vi "ADCP_read_symbol_file.vi"(8 "error in (no error)":errorcluster, 10 "Symbol File Path":path, 11 "ADCP in":refnum<class "ADCP.lvclass">) -> (0 "error out":errorcluster, 1 "Data Packets":T2(array[cluster]), 2 "Parameters":T3(array[cluster]), 3 "ADCP out":refnum<class "ADCP.lvclass">)   [LabVIEW 2017, in "ADCP.lvclass"]
uses:
  ADCP.lvclass
  ADCP_Data_Packet_Transmit_Mode.ctl
  ADCP.lvclass/ADCP.ctl
  <vilib>/Utility/file.llb/Read Delimited Spreadsheet (string).vi
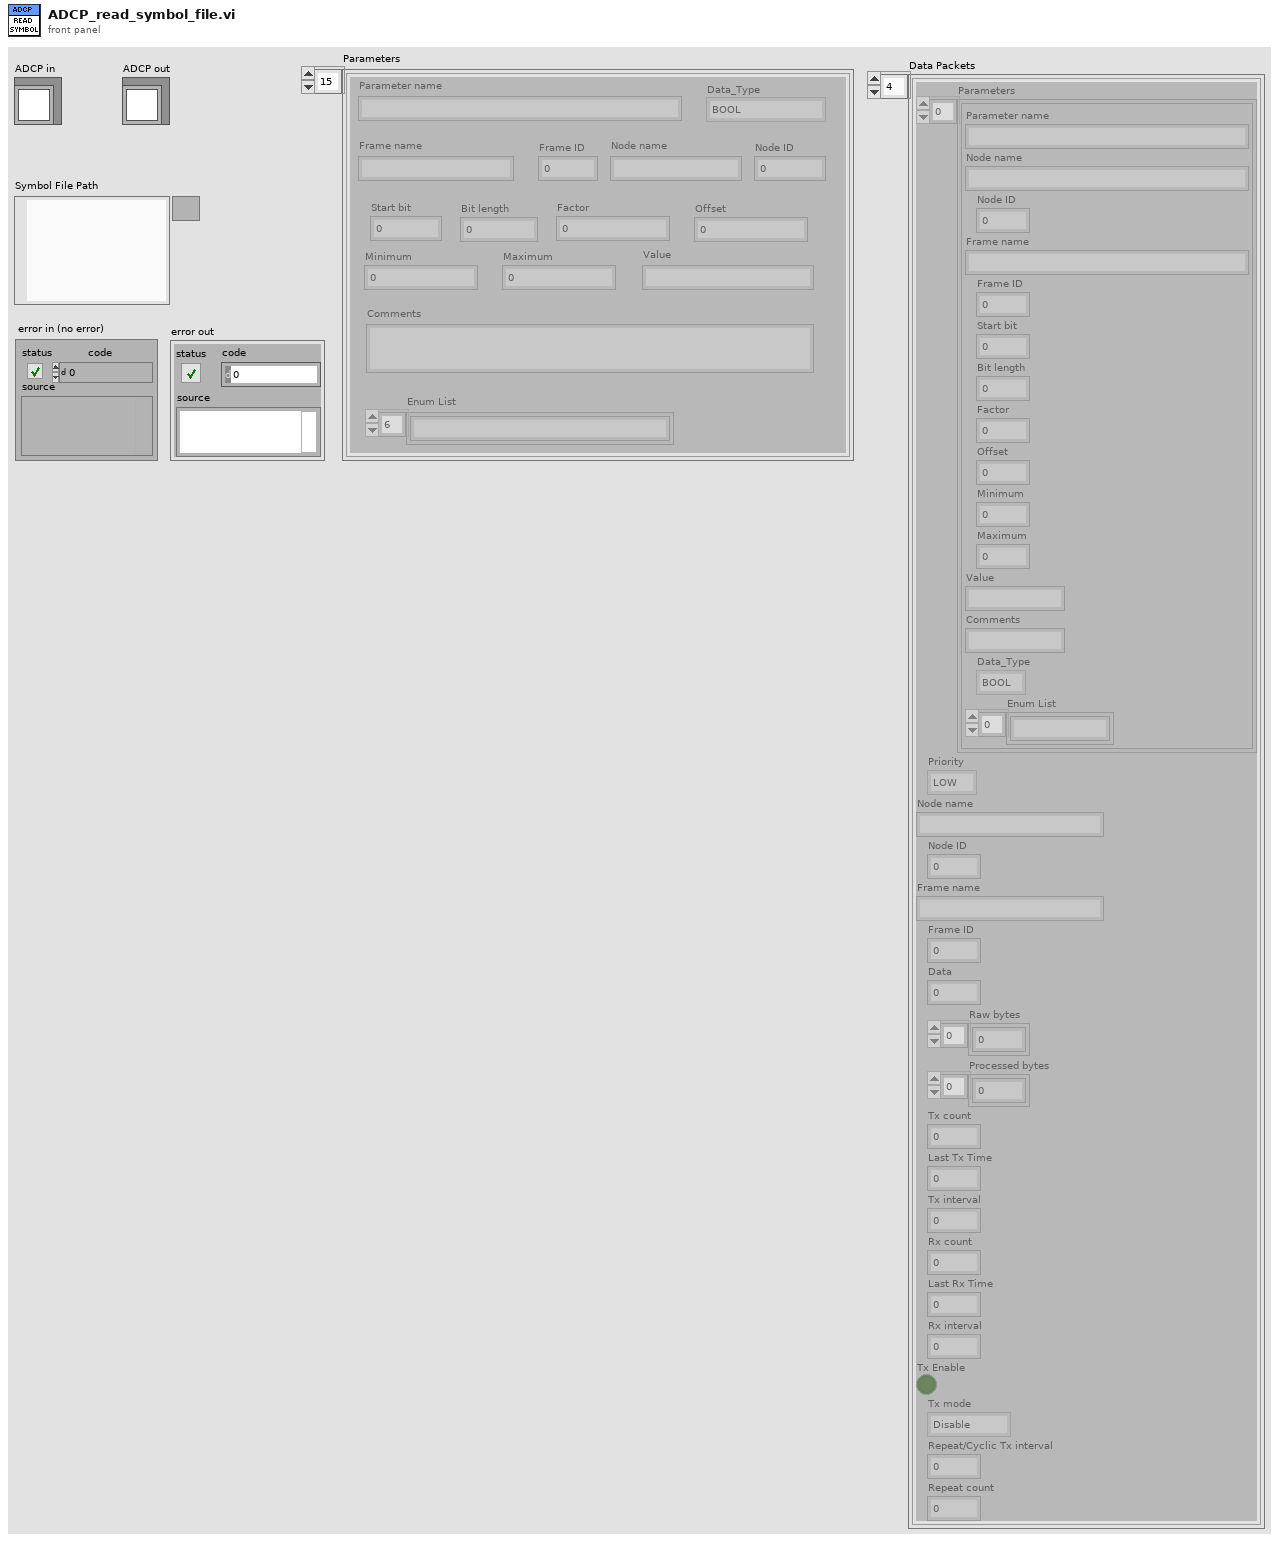
[diagram p1: front panel]
types:
  T1 = typedef "ADCP.lvclass/ADCP_Data_Packet_Transmit_Mode.ctl" = enum16{"Disable", "Single", "Cyclic", "Repeat"}
  T2 = cluster{"Parameters":cluster{"Parameter name":string, "Node name":string, "Node ID":u8, "Frame name":string, "Frame ID":u8, "Start bit":u32, "Bit length":u32, "Factor":dbl, "Offset":dbl, "Minimum":dbl, "Maximum":dbl, "Value":string, "Comments":string, "Data_Type":enum16{"BOOL", "UNSIGNED", "SIGNED", "FLOAT32", "ENUM"}, "Enum List":string[]}[], "Priority":enum16{"LOW", "HIGH"}, "Node name":string, "Node ID":u8, "Frame name":string, "Frame ID":u8, "Data":u32, "Raw bytes":u8[], "Processed bytes":u8[], "Tx count":i32, "Last Tx Time":u32, "Tx interval":u32, "Rx count":i32, "Last Rx Time":u32, "Rx interval":u32, "Tx Enable":bool, "Tx mode":T1, "Repeat/Cyclic Tx interval":u32, "Repeat count":u16}[]
  T3 = cluster{"Parameter name":string, "Node name":string, "Node ID":u8, "Frame name":string, "Frame ID":u8, "Start bit":u32, "Bit length":u32, "Factor":dbl, "Offset":dbl, "Minimum":dbl, "Maximum":dbl, "Value":string, "Comments":string, "Data_Type":enum16{"BOOL", "UNSIGNED", "SIGNED", "FLOAT32", "ENUM"}, "Enum List":string[]}[]
  T4 = cluster{"Parameter name":string, "Node name":string, "Node ID":u8, "Frame name":string, "Frame ID":u8, "Start bit":u32, "Bit length":u32, "Factor":dbl, "Offset":dbl, "Minimum":dbl, "Maximum":dbl, "Value":string, "Comments":string, "Data_Type":enum16{"BOOL", "UNSIGNED", "SIGNED", "FLOAT32", "ENUM"}, "Enum List":string[]}
  T5 = enum16{"BOOL", "UNSIGNED", "SIGNED", "FLOAT32", "ENUM"}
  T6 = cluster{"Parameters":cluster{"Parameter name":string, "Node name":string, "Node ID":u8, "Frame name":string, "Frame ID":u8, "Start bit":u32, "Bit length":u32, "Factor":dbl, "Offset":dbl, "Minimum":dbl, "Maximum":dbl, "Value":string, "Comments":string, "Data_Type":enum16{"BOOL", "UNSIGNED", "SIGNED", "FLOAT32", "ENUM"}, "Enum List":string[]}[], "Priority":enum16{"LOW", "HIGH"}, "Node name":string, "Node ID":u8, "Frame name":string, "Frame ID":u8, "Data":u32, "Raw bytes":u8[], "Processed bytes":u8[], "Tx count":i32, "Last Tx Time":u32, "Tx interval":u32, "Rx count":i32, "Last Rx Time":u32, "Rx interval":u32, "Tx Enable":bool, "Tx mode":T1, "Repeat/Cyclic Tx interval":u32, "Repeat count":u16}
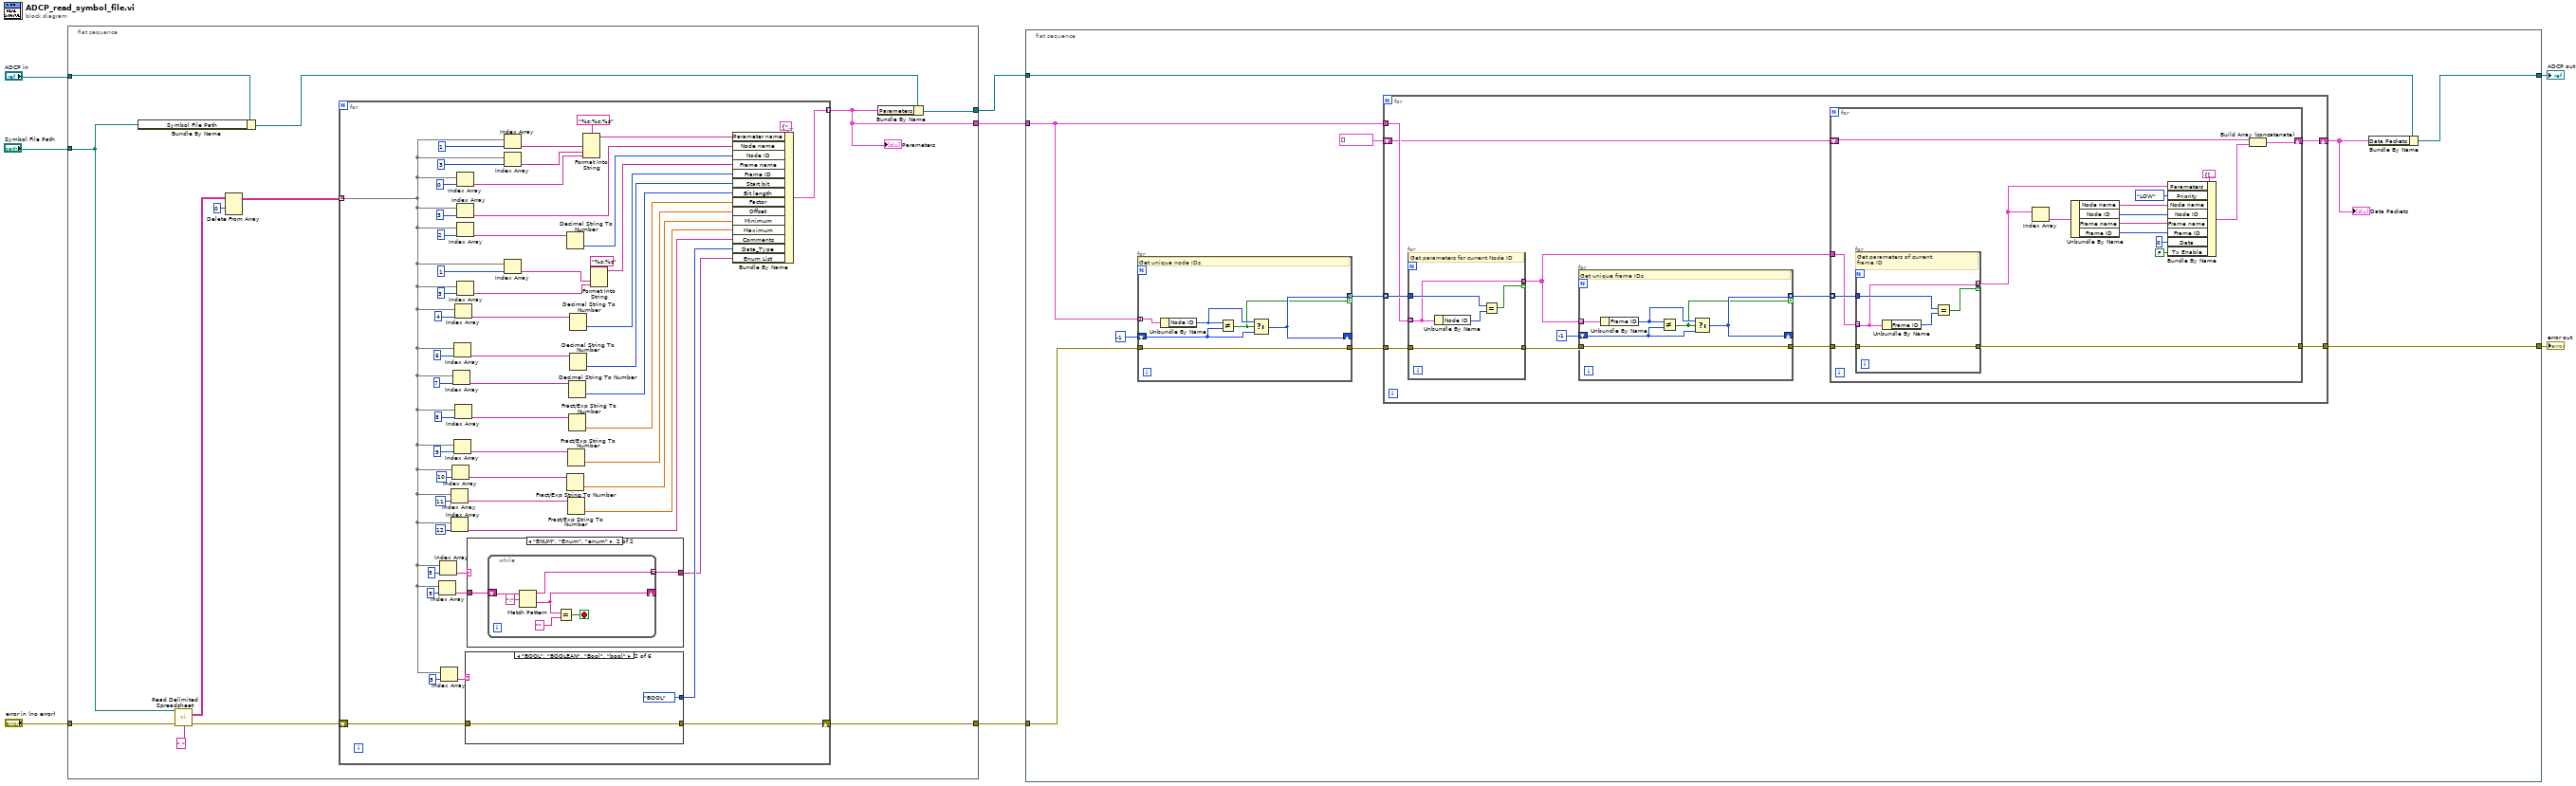
[diagram p0: block diagram]
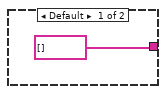
[diagram p2: hidden frame]
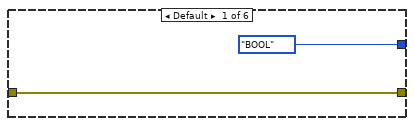
[diagram p3: hidden frame]
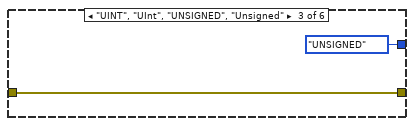
[diagram p4: hidden frame]
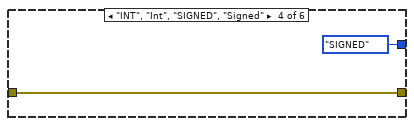
[diagram p5: hidden frame]
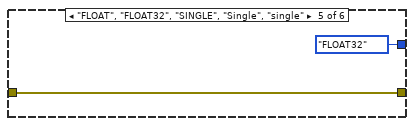
[diagram p6: hidden frame]
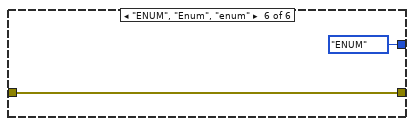
[diagram p7: hidden frame]
diagram:
  n1 = flat-sequence {
    tunnel: "Symbol File Path" -> [w11]
    tunnel: "error in (no error)" -> [w20]
    tunnel: "ADCP in" -> [w10]
    tunnel: [w18] -> w4
    tunnel: [w13] -> w5
    tunnel: [w12] -> w3
    frame #0 {
      n2 = Bundle By Name(cluster=w10, "Symbol File Path"=w11) -> (w9:refnum<class "ADCP.lvclass">)
      n3 = call-poly <vilib>:"Read Delimited Spreadsheet.vi"("file path (dialog if empty)"=w11, "error in (no error)"=w20, "delimiter (\\t)"="," ("delimiter (\\t)")) -> ("all rows"=w15:string[][], "error out"=w19:errorcluster)  [unwired: 7 in, 4 out]
      n4 = Delete From Array(array=w15, index (row)=0) -> (array with subset deleted=w14:string[][])  [unwired: 2 in, 1 out]
      n5 = for {
        shift-right: [w31] -> w13
        shift-left: w19 -> [w32]
        tunnel: w14 -> [w23] mode=indexing
        tunnel: [w21] -> w12 mode=indexing
        n6 = Index Array(array=w23, index=9) -> (element=w22:string)
        n7 = Index Array(array=w23, index=5) -> (element=w27:string)
        n8 = Index Array(array=w23, index=5) -> (element=w30:string)
        n9 = Index Array(array=w23, index=11) -> (element=w37:string)
        n10 = Index Array(array=w23, index=12) -> (element=w34:string)
        n11 = Index Array(array=w23, index=10) -> (element=w40:string)
        n12 = Index Array(array=w23, index=7) -> (element=w49:string)
        n13 = Index Array(array=w23, index=6) -> (element=w52:string)
        n14 = Index Array(array=w23, index=9) -> (element=w43:string)
        n15 = Index Array(array=w23, index=8) -> (element=w46:string)
        n16 = Index Array(array=w23, index=4) -> (element=w55:string)
        n17 = Index Array(array=w23, index=0) -> (element=w69:string)
        n18 = Index Array(array=w23, index=3) -> (element=w66:string)
        n19 = Index Array(array=w23, index=2) -> (element=w64:string)
        n20 = Index Array(array=w23, index=3) -> (element=w58:string)
        n21 = case shown="\"BOOL\", \"BOOLEAN\", \"Bool\", \"bool\"" w30 {
          tunnel: w32 -> [w86 w88 w90 w92 w94 w96]
          tunnel: [w86 w88 w90 w92 w94 w96] -> w31
          tunnel: [T5."BOOL" ("ADCP_Parameter_Data_Type") T5."BOOL" ("ADCP_Parameter_Data_Type") T5."UNSIGNED" ("ADCP_Parameter_Data_Type") T5."SIGNED" ("ADCP_Parameter_Data_Type") T5."FLOAT32" ("ADCP_Parameter_Data_Type") T5."ENUM" ("ADCP_Parameter_Data_Type")] -> w29
          frame Default {
          }
          frame "BOOL", "BOOLEAN", "Bool", "bool" {
          }
          frame "UINT", "UInt", "UNSIGNED", "Unsigned" {
          }
          frame "INT", "Int", "SIGNED", "Signed" {
          }
          frame "FLOAT", "FLOAT32", "SINGLE", "Single", "single" {
          }
          frame "ENUM", "Enum", "enum" {
          }
        }
        n22 = case shown="\"ENUM\", \"Enum\", \"enum\"" w27 {
          tunnel: [string[] [] w77] -> w25
          tunnel: w22 -> [_ w78]
          frame Default {
          }
          frame "ENUM", "Enum", "enum" {
            n23 = while {
              shift-right: [w81] -> _
              shift-left: w78 -> [w84]
              tunnel: [w80] -> w77 mode=indexing
              stop <- w82 stop-if-true
              n24 = Match Pattern(string=w84, regular expression=":") -> (before substring=w80:string, after substring=w81:string)  [unwired: 1 in, 2 out]
              n25 = Equal?(x=w81, y="") -> (x = y?=w82:bool)
            }
          }
        }
        n26 = Index Array(array=w23, index=3) -> (element=w71:string)
        n27 = Index Array(array=w23, index=1) -> (element=w59:string)
        n28 = Index Array(array=w23, index=1) -> (element=w73:string)
        n29 = Decimal String To Number(string=w64) -> (number=w63:i32)  [unwired: 2 in, 1 out]
        n30 = Fract/Exp String To Number(string=w40) -> (number=w39:dbl)  [unwired: 3 in, 1 out]
        n31 = Fract/Exp String To Number(string=w43) -> (number=w42:dbl)  [unwired: 3 in, 1 out]
        n32 = Fract/Exp String To Number(string=w37) -> (number=w36:dbl)  [unwired: 3 in, 1 out]
        n33 = Fract/Exp String To Number(string=w46) -> (number=w45:dbl)  [unwired: 3 in, 1 out]
        n34 = Decimal String To Number(string=w49) -> (number=w48:i32)  [unwired: 2 in, 1 out]
        n35 = Decimal String To Number(string=w52) -> (number=w51:i32)  [unwired: 2 in, 1 out]
        n36 = Decimal String To Number(string=w55) -> (number=w54:i32)  [unwired: 2 in, 1 out]
        n37 = Format Into String(format string="%s:%s:%s", w73, w71, w69) -> (resulting string=w68:string)  [unwired: 2 in, 1 out]
        n38 = Format Into String(format string="%s:%s", w59, w58) -> (resulting string=w57:string)  [unwired: 2 in, 1 out]
        n39 = Bundle By Name(cluster=T4 {"Parameter name"="", "Node name"="", "Node ID"=0, "Frame name"="", "Frame ID"=0, "Start bit"=0, "Bit length"=0, "Factor"=0.0, "Offset"=0.0, "Minimum"=0.0, "Maximum"=0.0, "Value"="", "Comments"="", "Data_Type"=enum."SIGNED", "Enum List"=[]} ("ADCP Parameter"), "Parameter name"=w68, "Node name"=w66, "Node ID"=w63, "Frame name"=w57, "Frame ID"=w54, "Start bit"=w51, "Bit length"=w48, "Factor"=w45, "Offset"=w42, "Minimum"=w39, "Maximum"=w36, "Comments"=w34, "Data_Type"=w29, "Enum List"=w25) -> (w21:T4)
      }
      "Parameters" <- w12
      n40 = Bundle By Name(cluster=w9, "Parameters"=w12) -> (w18:refnum<class "ADCP.lvclass">)
    }
  }
  n41 = flat-sequence {
    tunnel: w5 -> [w105]
    tunnel: w4 -> [w98]
    tunnel: w3 -> [w102]
    tunnel: [w100] -> w1
    tunnel: [w97] -> w2
    frame #0 {
      n42 = for {
        tunnel: w105 -> [w151]
        shift-right: [w153] -> _
        shift-left: -1 -> [w156]
        tunnel: w102 -> [w155] mode=indexing
        tunnel: [w153] -> w103 mode=indexing if=w152
        tunnel: [w151] -> w104
        # "Get unique node IDs"
        n43 = Unbundle By Name(w155) -> ("Node ID"=w154:u8)
        n44 = Not Equal?(x=w154, y=w156) -> (x != y?=w152:bool)
        n45 = Select(t=w154, s=w152, f=w156) -> (s? t:f=w153:i32)
      }
      n46 = for {
        tunnel: w104 -> [w117]
        tunnel: w103 -> [w116] mode=indexing
        tunnel: w102 -> [w115]
        shift-right: [w108] -> w99
        shift-left: T2 [] -> [w109]
        tunnel: [w107] -> w100
        n47 = for {
          tunnel: w117 -> [w148]
          tunnel: w116 -> [w150]
          tunnel: w115 -> [w147] mode=indexing
          tunnel: [w148] -> w113
          tunnel: [w147] -> w110 mode=indexing if=w146
          # "Get parameters for current Node ID"
          n48 = Unbundle By Name(w147) -> ("Node ID"=w149:u8)
          n49 = Equal?(x=w150, y=w149) -> (x = y?=w146:bool)
        }
        n50 = for {
          tunnel: w113 -> [w140]
          shift-right: [w142] -> _
          shift-left: -1 -> [w145]
          tunnel: w110 -> [w144] mode=indexing
          tunnel: [w142] -> w111 mode=indexing if=w141
          tunnel: [w140] -> w112
          # "Get unique frame IDs"
          n51 = Unbundle By Name(w144) -> ("Frame ID"=w143:u8)
          n52 = Not Equal?(x=w143, y=w145) -> (x != y?=w141:bool)
          n53 = Select(t=w143, s=w141, f=w145) -> (s? t:f=w142:i32)
        }
        n54 = for {
          tunnel: w112 -> [w134]
          tunnel: w111 -> [w133] mode=indexing
          tunnel: w110 -> [w132]
          tunnel: [w121] -> w107
          shift-right: [w119] -> w108
          shift-left: w109 -> [w120]
          n55 = for {
            tunnel: w134 -> [w135]
            tunnel: w133 -> [w139]
            tunnel: w132 -> [w137] mode=indexing
            tunnel: [w137] -> w129 mode=indexing if=w136
            tunnel: [w135] -> w121
            # "Get parameters of current\nframe ID"
            n56 = Unbundle By Name(w137) -> ("Frame ID"=w138:u8)
            n57 = Equal?(x=w139, y=w138) -> (x = y?=w136:bool)
          }
          n58 = Index Array(array=w129) -> (element=w128:T4)  [unwired: 1 in]
          n59 = Unbundle By Name(w128) -> ("Node name"=w127:string, "Node ID"=w126:u8, "Frame name"=w125:string, "Frame ID"=w124:u8)
          n60 = Bundle By Name(cluster=T6 {"Parameters"=[], "Priority"=enum."LOW", "Node name"="", "Node ID"=0, "Frame name"="", "Frame ID"=0, "Data"=0, "Raw bytes"=[], "Processed bytes"=[], "Tx count"=0, "Last Tx Time"=0, "Tx interval"=0, "Rx count"=0, "Last Rx Time"=0, "Rx interval"=0, "Tx Enable"=FALSE, "Tx mode"=enum."Disable", "Repeat/Cyclic Tx interval"=0, "Repeat count"=0} ("ADCP Data Packet"), "Parameters"=w129, "Priority"=enum16{"LOW", "HIGH"}."LOW", "Node name"=w127, "Node ID"=w126, "Frame name"=w125, "Frame ID"=w124, "Data"=u32 0, "Tx Enable"=FALSE) -> (w118:T6)
          n61 = Build Array (concatenate)(w120, w118) -> (w119:T2)
        }
      }
      "Data Packets" <- w99
      n62 = Bundle By Name(cluster=w98, "Data Packets"=w99) -> (w97:refnum<class "ADCP.lvclass">)
    }
  }
  "ADCP out" <- w2
  "error out" <- w1
